vi "setArmStimulus.vi"(8 "error in (no error)":errorcluster, 10 "channel":i32, 11 "K2602 in":refnum<class "K2602.lvclass">) -> (0 "error out":errorcluster, 3 "K2602 out":refnum<class "K2602.lvclass">)   [LabVIEW 2009, in "Hardware.lvlib" / "Channels.lvlib" / "K2602.lvclass"]
uses:
  K2602.lvclass
  K2602.lvclass/K2602.ctl
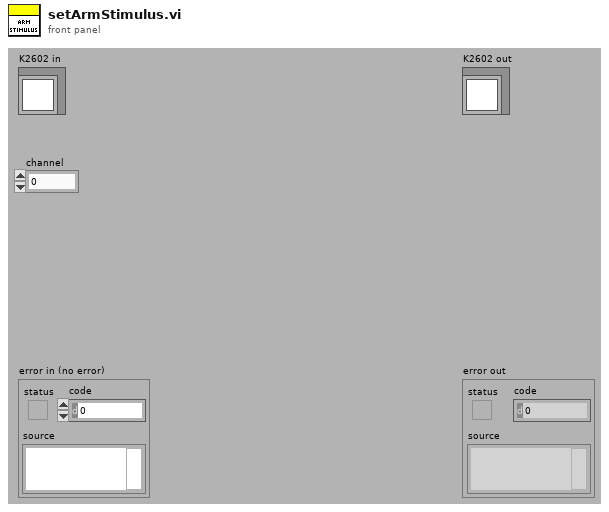
[diagram p1: front panel]
types:
  T1 = cluster{"Range":cluster{"current":dbl, "voltage":dbl}, "triggering_inUse":cluster{"start_trigger":string, "clock":string}, "Limits":cluster{"VoltageLimit":dbl, "CurrentLimit":dbl}}[]
  T2 = cluster{"Range":cluster{"current":dbl, "voltage":dbl}, "triggering_inUse":cluster{"start_trigger":string, "clock":string}, "Limits":cluster{"VoltageLimit":dbl, "CurrentLimit":dbl}}
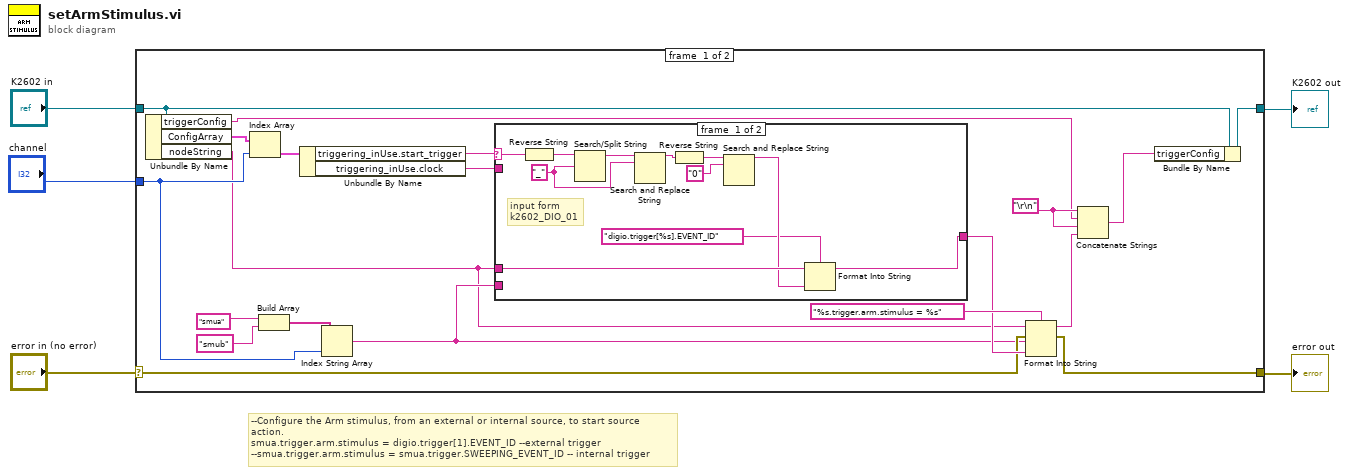
[diagram p0: block diagram]
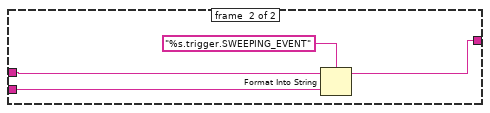
[diagram p2: hidden frame]
diagram:
  # "--Configure the Arm stimulus, from an external or internal source, to start source action.\nsmua.trigger.arm.stimulus = digio.trigger[1].EVENT_ID --external trigger\n--smua.trigger.arm.stimulus = smua.trigger.SWEEPING_EVENT_ID -- internal trigger"
  n1 = case shown="No Error" "error in (no error)" {
    selector: "error in (no error)" -> [w15 w42]
    tunnel: [w14 w42] -> w4
    tunnel: [w6 w41] -> w2
    tunnel: "K2602 in" -> [w8 w41]
    tunnel: "channel" -> [w18 _]
    frame #0 {
      w11 = "\r\n"
      n2 = Unbundle By Name(w8) -> ("triggerConfig"=w9:string, "ConfigArray"=w25:T1, "nodeString"=w12:string)
      n3 = Index Array(array=w25, index=w18) -> (element=w24:T2)
      n4 = Build Array("smua", "smub") -> (w19:string[])
      n5 = Unbundle By Name(w24) -> ("triggering_inUse.start_trigger"=w23:string, "triggering_inUse.clock"=w22:string)
      n6 = Index String Array(1:w18, 2:w19) -> (0:w13:string)  [unwired: 1 in]
      n7 = case shown="Default" w23 {
        selector: w23 -> [w36 _]
        tunnel: w22 -> [_ _]
        tunnel: w12 -> [w29 w40]
        tunnel: [w26 w37] -> w16
        tunnel: w13 -> [_ w39]
        frame #0 {
          w33 = "_"
          # "input form\nk2602_DIO_01"
          n8 = Reverse String(1:w36) -> (0:w35:string)
          n9 = Search/Split String(string=w35, search string/char (-)=w33) -> (substring before match=w34:string)  [unwired: 1 in, 2 out]
          n10 = Search and Replace String(input string=w34, search string=w33) -> (result string=w32:string)  [unwired: 6 in, 3 out]
          n11 = Reverse String(1:w32) -> (0:w31:string)
          n12 = Search and Replace String(input string=w31, search string="0") -> (result string=w28:string)  [unwired: 6 in, 3 out]
          n13 = Format Into String(format string="digio.trigger[%s].EVENT_ID", initial string=w29, w28) -> (resulting string=w26:string)  [unwired: 1 in, 1 out]
        }
        frame #1 {
          n14 = Format Into String(format string="%s.trigger.SWEEPING_EVENT", initial string=w40, w39) -> (resulting string=w37:string)  [unwired: 1 in, 1 out]
        }
      }
      n15 = Format Into String(format string="%s.trigger.arm.stimulus = %s", initial string=w12, error in=w15, w13, w16) -> (resulting string=w10:string, error out=w14:errorcluster)
      n16 = Concatenate Strings(w11, w9, w11, w10) -> (w7:string)
      n17 = Bundle By Name(cluster=w8, "triggerConfig"=w7) -> (w6:refnum<class "K2602.lvclass">)
    }
    frame #1 {
    }
  }
  "error out" <- w4
  "K2602 out" <- w2
